vi "Mouseclick.vi"(9 "nMilliseconds":i32=2000, 10 "error in (no error)":errorcluster) -> (2 "error out":errorcluster)   [LabVIEW 2014]
panel:
  in  "AutoItX3Lib.IAutoItX3":refnum<k7>
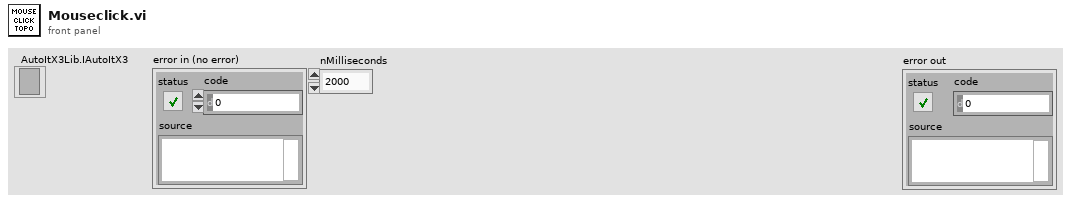
[diagram p1: front panel]
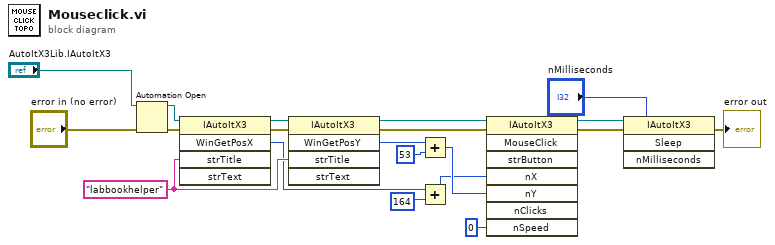
[diagram p0: block diagram]
diagram:
  w14 = "labbookhelper" ("strTitle")
  n1 = Automation Open(error in (no error)="error in (no error)", Automation Refnum="AutoItX3Lib.IAutoItX3") -> (Automation Refnum=w16:refnum<k7>, error out=w17:errorcluster)  [unwired: 2 in]
  n2 = invoke class="IAutoItX3" method="WinGetPosX"(reference=w16, error in=w17, "strTitle"=w14) -> (reference out=w12:refnum<k7>, error out=w13:errorcluster, "WinGetPosX"=w10:i32)  [unwired: 2 in, 2 out]
  n3 = invoke class="IAutoItX3" method="WinGetPosY"(reference=w12, error in=w13, "strTitle"=w14) -> (reference out=w19:refnum<k7>, error out=w18:errorcluster, "WinGetPosY"=w11:i32)  [unwired: 2 in, 2 out]
  n4 = Add(x=w11, y=53) -> (x+y=w9:i32)
  n5 = Add(x=w10, y=164) -> (x+y=w5:i32)
  n6 = invoke class="IAutoItX3" method="MouseClick"(reference=w19, error in=w18, "nX"=w5, "nY"=w9, "nSpeed"=0) -> (reference out=w7:refnum<k7>, error out=w6:errorcluster)  [unwired: 3 in, 6 out]
  n7 = invoke class="IAutoItX3" method="Sleep"(reference=w7, error in=w6, "nMilliseconds"="nMilliseconds") -> (error out=→"error out":errorcluster)  [unwired: 1 in, 3 out]
